vi "SetSyncOffset.vi"(8 "error in (no error)":errorcluster, 10 "Offset":i32, 11 "Multiharp in":refnum<class "Multiharp.lvclass">) -> (0 "error out":errorcluster, 3 "Multiharp out":refnum<class "Multiharp.lvclass">)   [LabVIEW 2023, in "Multiharp.lvlib" / "Multiharp.lvclass"]
uses:
  Multiharp.lvclass
  <vilib>/ActorFramework/Actor/Actor.lvclass
  Multiharp Messages/SetSyncDeadTime Msg/SetSyncDeadTime Msg.lvclass
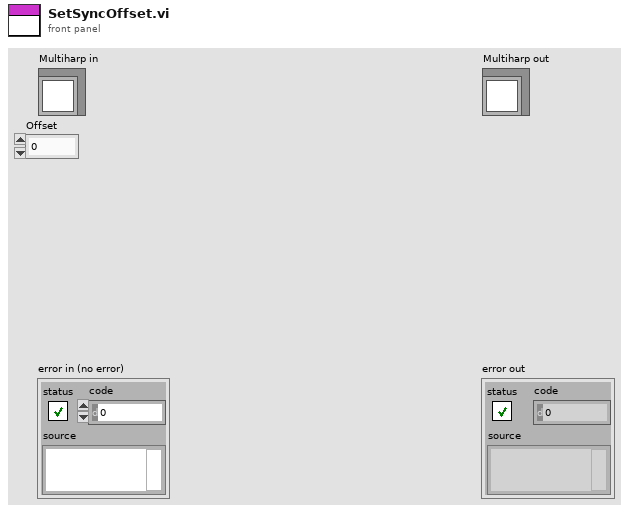
[diagram p1: front panel]
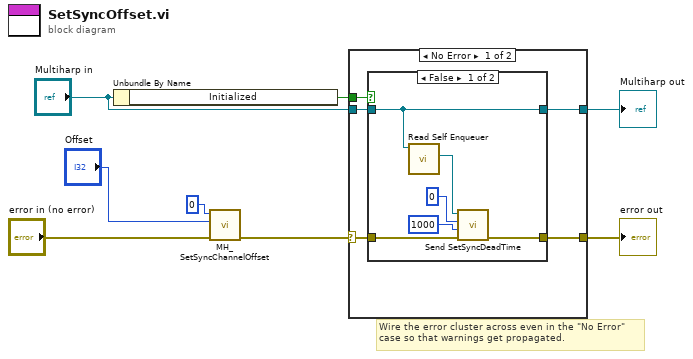
[diagram p0: block diagram]
diagram:
  # "Wire the error cluster across even in the \"No Error\"\ncase so that warnings get propagated."
  n1 = Unbundle By Name("Multiharp in") -> ("Initialized"=w8:bool)
  n2 = call "MH_SetSyncChannelOffset.vi"("error in (no error)"="error in (no error)", "Offset"="Offset", "devidx"=0) -> ("error out"=w6:errorcluster)  [unwired: 7 in, 1 out]
  n3 = case shown="No Error" w6 {
    selector: w6 -> [w10 w22]
    tunnel: w8 -> [w13 _]
    tunnel: "Multiharp in" -> [w12 w23]
    tunnel: [w11 w23] -> w2
    tunnel: [w9 w22] -> w4
    frame No Error {
      n4 = case shown="False" w13 {
        tunnel: w12 -> [w19 w21]
        tunnel: [w19 w21] -> w11
        tunnel: w10 -> [w15 w20]
        tunnel: [w14 w20] -> w9
        frame False {
          n5 = call <vilib>:"Read Self Enqueuer.vi"("Actor"=w19) -> ("Self Enqueuer"=w18:refnum<class "Message Enqueuer.lvclass">)  [unwired: 10 in]
          n6 = call "Send SetSyncDeadTime.vi"("error in (no error)"=w15, "deadtime"=1000, "on"=0, "Message Enqueuer"=w18) -> ("error out"=w14:errorcluster)  [unwired: 6 in, 1 out]
        }
        frame True {
          # "Send message to UI"
        }
      }
    }
    frame Error {
    }
  }
  "error out" <- w4
  "Multiharp out" <- w2
